vi "NI 5433 (Host)_Independent.vi"() -> ()   [LabVIEW 2020]
uses:
  <instrlib>/niFgen/niFgen.llb/niFgen Output Mode.ctl
  <instrlib>/niFgen/niFgen.llb/niFgen_ctl Trigger SW - TrigName Values (Ring).ctl
  <instrlib>/niFgen/niFgen.llb/niFgen Trigger Mode.ctl
  <instrlib>/niFgen/niFgen.llb/niFgen Configure Software Edge Start Trigger.vi
  <instrlib>/niFgen/niFgen.llb/niFgen Configure Digital Edge Start Trigger.vi
  <instrlib>/niFgen/niFgen.llb/niFgen Disable Start Trigger.vi
  <instrlib>/niFgen/niFgen.llb/niFgen Create Waveform (DBL).vi
  <instrlib>/niFgen/niFgen.llb/niFgen_ctl Exported Signal Name Values (Ring).ctl
  <instrlib>/niFgen/niFgen.llb/niFgen_ctl Exported Signal Identifiers (Ring).ctl
panel:
  in  "Wave Per Pixel":i32
  in  "Source (PFI 0)":string(combo)="PXI_Trig1" caption="Trigger Source"
  in  "Trigger Type":u16(ring)=2 items=["None", "Software Edge", "Digital Edge"]
  in  "Send Software Trigger":bool
  in  "FGEN Resource Name":refnum<k15>
  in  "Stop":bool
  in  "Update":bool
  in  "Analog Filter":bool
  in  "Digital Filter":bool
  in  "Gain":dbl(knob)=1.0 min=0.0 max=5.0 scale=0.0..5.0 scale format="%#.1f"
  in  "Sample Rate (S/s)":dbl=200000000.0 format="%.2p"
  in  "DC Offset (V)":dbl(knob) scale=-0.5..0.5 scale format="%#.1f"
  in  "Waveform Information Array":T1(array[cluster])=[{"Waveform Type"=0, "Amplitude"=1.0, "# of points"=256}] {"Amplitude" min=0.0 max=1.0 format="%.2f"; "Waveform Type" items=["Sine", "Cosine", "Triangle", "Square", "Sawtooth", "Increasing Ramp", "Decreasing Ramp", "DC Value"]}
  out "Actual Sample Rate (S/s)":dbl format="%.2p"
  out "Waveform Graph":dbl[](graph)
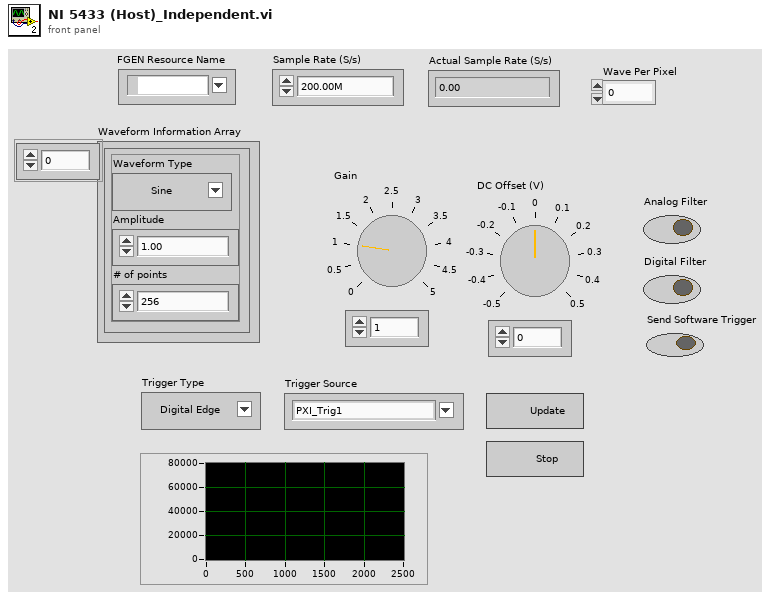
[diagram p1: front panel]
types:
  T1 = cluster{"Waveform Type":u16, "Amplitude":dbl, "# of points":u32}[]
  T2 = typedef "niFgen_ctl Exported Signal Identifiers (Ring).ctl" = string
  T3 = typedef "niFgen_ctl Exported Signal Name Values (Ring).ctl" = u16
  T4 = typedef "niFgen Trigger Mode.ctl" = i32
  T5 = typedef "niFgen Output Mode.ctl" = u32
  T6 = typedef "niFgen_ctl Trigger SW - TrigName Values (Ring).ctl" = i32
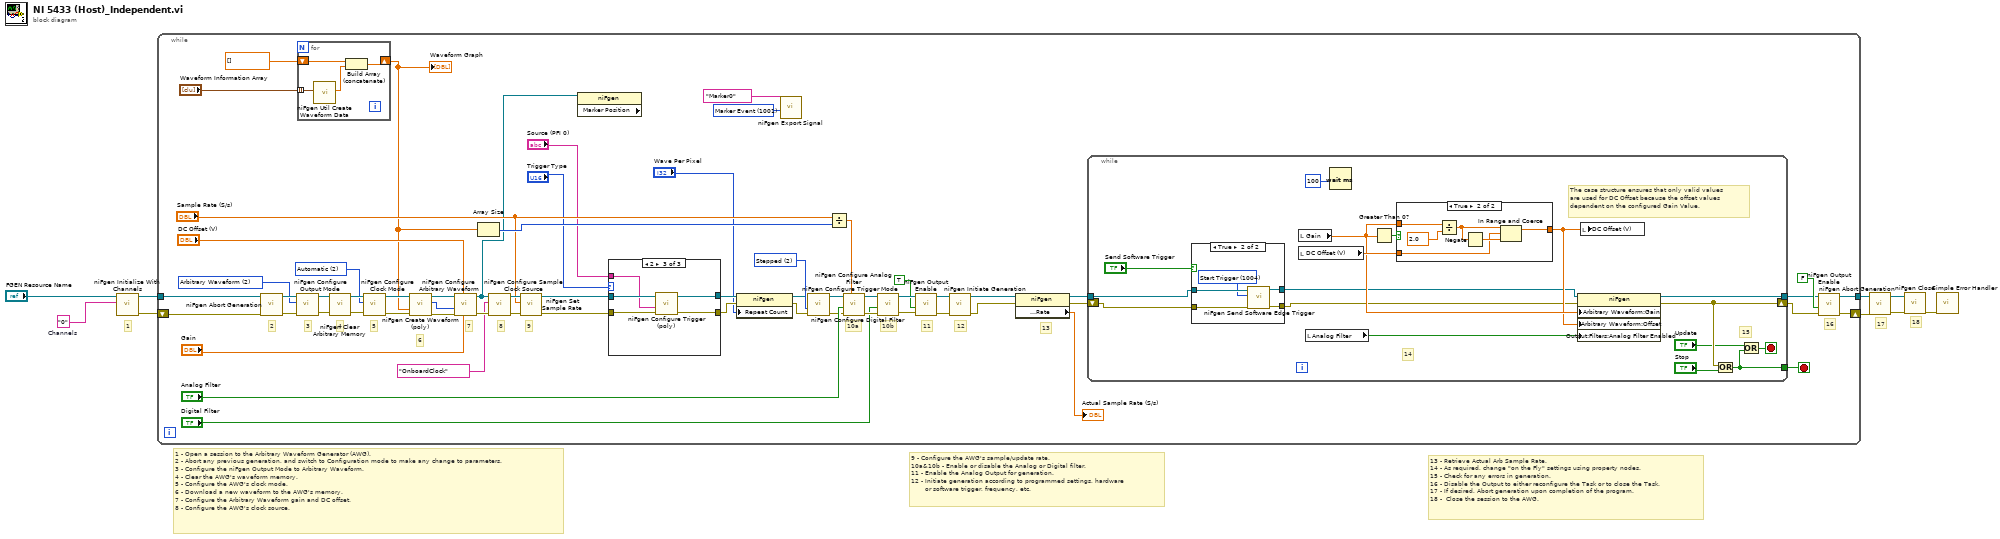
[diagram p0: block diagram]
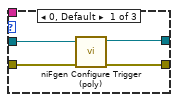
[diagram p2: hidden frame]
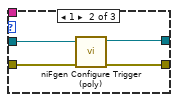
[diagram p3: hidden frame]
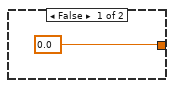
[diagram p5: hidden frame]
diagram:
  w3 = "0"  # Channels
  # "9 - Configure the AWG's sample/update rate.\n10a&10b - Enable or disable the Analog or Digital filter.\n11 - Enable the Analog Output for generation.\n12 - Initiate generation according to programmed settings, hardware\n       or software trigger, frequency, etc."
  # "18"
  # "17"
  # "1"
  # "1 - Open a session to the Arbitrary Waveform Generator (AWG).\n2 - Abort any previous generation, and switch to Configuration mode to make any change to parameters.\n3 - Configure the niFgen Output Mode to Arbitrary Waveform.\n4 - Clear the AWG's waveform memory.\n5 - Configure the AWG's clock mode.\n6 - Download a new waveform to the AWG's memory.\n7 - Configure the Arbitrary Waveform gain and DC offset.\n8 - Configure the AWG's clock source."
  # "13 - Retrieve Actual Arb Sample Rate.\n14 - As required, change \"on the Fly\" settings using property nodes.\n15 - Check for any errors in generation.\n16 - Disable the Output to either reconfigure the Task or to close the Task. \n17 - If desired, Abort generation upon completion of the program.\n18 -  Close the session to the AWG."
  n1 = call <instrlib>:"niFgen Initialize With Channels.vi"("Channel Name"=w3, "Resource Name"="FGEN Resource Name") -> ("error out"=w2:errorcluster, "Instrument Handle Out"=w1:refnum<k15>)  [unwired: 8 in]
  n2 = while {
    tunnel: [w30] -> w9
    tunnel: w1 -> [w70]
    shift-right: [w26] -> w5
    shift-left: w2 -> [w46]
    stop <- w33 stop-if-true
    w12 = T3 1001 items=["Sample Clock"=101, "Sample Clock Timebase"=1006, "Reference Clock"=102, "Onboard Reference Clock"=1019, "Start Trigger"=1004, "Script Trigger"=103, "Marker Event"=1001, "Data Marker Event"=108, "Ready For Start Event"=105, "Started Event"=106, "Done Event"=107, "Synchronization Pulse"=1007, "Sync Out"=1002] ("Signal")
    w37 = u32 2 items=["Hi Resolution Sampling", "Divide Down Sampling", "Automatic"] ("Clock Mode")
    w23 = T4 2 items=["Single", "Continuous", "Stepped", "Burst"] ("Trigger Mode (default: 1=continuous)")
    w60 = T5 2 items=["Standard Function", "Frequency List", "Arbitrary Waveform", "Arbitrary Sequence", "Script"] ("Output Mode")
    # "16"
    # "12"
    # "11"
    # "10b"
    # "10a"
    # "9"
    # "8"
    # "7"
    # "6"
    # "5"
    # "4"
    # "3"
    # "2"
    # "13"
    n3 = call <instrlib>:"niFgen Abort Generation.vi"("error in (no error)"=w46, "Instrument Handle"=w70) -> ("error out"=w67:errorcluster, "Instrument Handle Out"=w66:refnum<k15>)  [unwired: 8 in]
    n4 = call <instrlib>:"niFgen Configure Output Mode.vi"("error in (no error)"=w67, "Output Mode (default: 0=Standard Function)"=w60, "Instrument Handle"=w66) -> ("error out"=w56:errorcluster, "Instrument Handle Out"=w59:refnum<k15>)  [unwired: 6 in]
    n5 = for {
      shift-right: [w116] -> w18
      shift-left: dbl[] [] -> [w119]
      tunnel: "Waveform Information Array" -> [w117] mode=indexing
      n6 = call <instrlib>:"niFgen Util Create Waveform Data.vi"("Waveform"=w117) -> ("Waveform Data"=w118:dbl[])  [unwired: 10 in]
      n7 = Build Array (concatenate)(w119, w118) -> (w116:dbl[])
    }
    "Waveform Graph" <- w18
    n8 = call <instrlib>:"niFgen Clear Arbitrary Memory.vi"("error in (no error)"=w56, "Instrument Handle"=w59) -> ("error out"=w57:errorcluster, "Instrument Handle Out"=w58:refnum<k15>)  [unwired: 8 in]
    n9 = call <instrlib>:"niFgen Configure Clock Mode.vi"("error in (no error)"=w57, "Clock Mode (default: 1=divide down)"=w37, "Instrument Handle"=w58) -> ("error out"=w64:errorcluster, "Instrument Handle Out"=w65:refnum<k15>)  [unwired: 7 in]
    n10 = call-poly <instrlib>:"niFgen Create Waveform (poly).vi"("error in (no error)"=w64, "Waveform Data Array"=w18, "Instrument Handle"=w65) -> ("error out"=w68:errorcluster, "Waveform Handle"=w27:i32, "Instrument Handle Out"=w69:refnum<k15>)  [unwired: 6 in]
    n11 = call <instrlib>:"niFgen Configure Arbitrary Waveform.vi"("Gain"="Gain", "Offset"="DC Offset (V)", "error in (no error)"=w68, "Waveform Handle"=w27, "Instrument Handle"=w69) -> ("error out"=w63:errorcluster, "Instrument Handle Out"=w10:refnum<k15>)  [unwired: 5 in]
    n12 = Array Size(array=w18) -> (size(s)=w48:i32)
    n13 = call <instrlib>:"niFgen Configure Sample Clock Source.vi"("error in (no error)"=w63, "Source (Onboard Clock)"="OnboardClock" ("Sample Clock Source"), "Instrument Handle"=w10) -> ("error out"=w54:errorcluster, "Instrument Handle Out"=w55:refnum<k15>)  [unwired: 7 in]
    n14 = call <instrlib>:"niFgen Set Sample Rate.vi"("error in (no error)"=w54, "Sample Rate (Samp/s)"="Sample Rate (S/s)", "Instrument Handle"=w55) -> ("error out"=w19:errorcluster, "Instrument Handle Out"=w20:refnum<k15>)  [unwired: 7 in]
    n15 = property class="niFgen" props=["Marker Position"](reference=w10) -> ()  [unwired: 1 in, 3 out]
    n16 = case shown="2" "Trigger Type" {
      tunnel: [w75 w79 w84] -> w15
      tunnel: w20 -> [w74 w78 w83]
      tunnel: w19 -> [w73 w77 w82]
      tunnel: [w72 w76 w81] -> w14
      tunnel: "Source (PFI 0)" -> [_ _ w80]
      frame 0, Default {
        n17 = call-poly <instrlib>:"niFgen Configure Trigger (poly).vi"("error in (no error)"=w73, "Instrument Handle"=w74) -> ("error out"=w72:errorcluster, "Instrument Handle Out"=w75:refnum<k15>)  [unwired: 8 in]
      }
      frame 1 {
        n18 = call-poly <instrlib>:"niFgen Configure Trigger (poly).vi"("error in (no error)"=w77, "Instrument Handle"=w78) -> ("error out"=w76:errorcluster, "Instrument Handle Out"=w79:refnum<k15>)  [unwired: 8 in]
      }
      frame 2 {
        n19 = call-poly <instrlib>:"niFgen Configure Trigger (poly).vi"("error in (no error)"=w82, "Source"=w80, "Instrument Handle"=w83) -> ("error out"=w81:errorcluster, "Instrument Handle Out"=w84:refnum<k15>)  [unwired: 7 in]
      }
    }
    n20 = property class="niFgen"(reference=w15, error in=w14, "Repeat Count"="Wave Per Pixel") -> (reference out=w17:refnum<k15>, error out=w16:errorcluster)
    n21 = call <instrlib>:"niFgen Export Signal.vi"("Signal"=w12, "Signal Identifier (None)"=T2 "Marker0") -> ()  [unwired: 8 in, 2 out]
    n22 = call <instrlib>:"niFgen Configure Trigger Mode.vi"("error in (no error)"=w16, "Trigger Mode (default: 1=continuous)"=w23, "Instrument Handle"=w17) -> ("error out"=w24:errorcluster, "Instrument Handle Out"=w25:refnum<k15>)  [unwired: 7 in]
    n23 = Divide(x="Sample Rate (S/s)", y=w48) -> (x/y=w49:dbl)
    n24 = call <instrlib>:"niFgen Configure Analog Filter.vi"("Filter Correction Frequency"=w49, "error in (no error)"=w24, "Analog Filter Enable (default: True)"="Analog Filter", "Instrument Handle"=w25) -> ("error out"=w53:errorcluster, "Instrument Handle Out"=w52:refnum<k15>)  [unwired: 6 in]
    n25 = call <instrlib>:"niFgen Configure Digital Filter.vi"("error in (no error)"=w53, "Digital Filter Enable (default: True)"="Digital Filter", "Instrument Handle"=w52) -> ("error out"=w50:errorcluster, "Instrument Handle Out"=w51:refnum<k15>)  [unwired: 7 in]
    n26 = call <instrlib>:"niFgen Output Enable.vi"("error in (no error)"=w50, "Output Enable (default: True)"=TRUE ("output enable"), "Instrument Handle"=w51) -> ("error out"=w61:errorcluster, "Instrument Handle Out"=w62:refnum<k15>)  [unwired: 7 in]
    n27 = call <instrlib>:"niFgen Initiate Generation.vi"("error in (no error)"=w61, "Instrument Handle"=w62) -> ("error out"=w44:errorcluster, "Instrument Handle Out"=w45:refnum<k15>)  [unwired: 8 in]
    n28 = property class="niFgen"(reference=w45, error in=w44) -> (reference out=w43:refnum<k15>, error out=w42:errorcluster, "Clocks:Sample Clock:Rate"=→"Actual Sample Rate (S/s)":dbl)
    n29 = while {
      tunnel: w43 -> [w88]
      tunnel: [w90] -> w33
      tunnel: [w91] -> w29
      shift-right: [w96] -> w31
      shift-left: w42 -> [w87]
      stop <- w99 stop-if-true
      # "The case structure ensures that only valid values \nare used for DC Offset because the offset values \ndependent on the configured Gain Value."
      # "15"
      # "14"
      n30 = case shown="True" "Send Software Trigger" {
        tunnel: w88 -> [w103 w108]
        tunnel: [w103 w107] -> w85
        tunnel: w87 -> [w102 w106]
        tunnel: [w102 w105] -> w86
        frame False {
        }
        frame True {
          w104 = T6 1004 items=["Start Trigger"=1004, "Script Trigger"=104] ("Trigger (Start Trigger)")
          n31 = call <instrlib>:"niFgen Send Software Edge Trigger.vi"("error in (no error)"=w106, "Trigger (Start Trigger)"=w104, "Instrument Handle"=w108) -> ("error out"=w105:errorcluster, "Instrument Handle Out"=w107:refnum<k15>)  [unwired: 7 in]
        }
      }
      n32 = local read "Gain"() -> (w97:dbl)
      n33 = local read "DC Offset (V)"() -> (w98:dbl)
      n34 = local read "Analog Filter"() -> (w92:bool)
      n35 = Wait (ms)(milliseconds to wait=u32 100 ("millisecond multiple")) -> ()  [unwired: 1 out]
      n36 = Greater Than 0?(x=w97) -> (x > 0?=w100:bool)
      n37 = case shown="True" w100 {
        tunnel: w97 -> [_ w114]
        tunnel: [0.0 ("DC Offset") w110] -> w93
        tunnel: w98 -> [_ w111]
        frame False {
        }
        frame True {
          n38 = Divide(x=w114, y=2.0) -> (x/y=w113:dbl)
          n39 = Negate(x=w113) -> (-x=w112:dbl)
          n40 = In Range and Coerce(upper limit=w113, x=w111, lower limit=w112) -> (coerced(x)=w110:dbl)  [unwired: 1 out]
        }
      }
      n41 = property class="niFgen"(reference=w85, error in=w86, "Arbitrary Waveform:Gain"=w97, "Arbitrary Waveform:Offset"=w93, "Output:Filters:Analog Filter Enabled"=w92) -> (reference out=w91:refnum<k15>, error out=w96:errorcluster)
      n42 = local write "DC Offset (V)"(w93) -> ()
      n43 = Or(x=w96, y="Stop") -> (x .or. y?=w90:bool)
      n44 = Or(x="Update", y=w90) -> (x .or. y?=w99:bool)
    }
    n45 = call <instrlib>:"niFgen Output Enable.vi"("error in (no error)"=w31, "Output Enable (default: True)"=FALSE ("output enable"), "Instrument Handle"=w29) -> ("error out"=w26:errorcluster, "Instrument Handle Out"=w30:refnum<k15>)  [unwired: 7 in]
  }
  n46 = call <instrlib>:"niFgen Abort Generation.vi"("error in (no error)"=w5, "Instrument Handle"=w9) -> ("error out"=w8:errorcluster, "Instrument Handle Out"=w7:refnum<k15>)  [unwired: 8 in]
  n47 = call <instrlib>:"niFgen Close.vi"("error in (no error)"=w8, "Instrument Handle"=w7) -> ("error out"=w6:errorcluster)  [unwired: 9 in]
  n48 = call <vilib>:"Simple Error Handler.vi"("error in (no error)"=w6) -> ()  [unwired: 4 in, 5 out]
